vi "HapticSTM-Height.vi"() -> ()   [LabVIEW 2019]
uses:
  <userlib>/HapticSTM/HapticSTM.lvlib
panel:
  out "ZVAL":dbl
  out "Target Z":dbl
  out "Target X":dbl
  out "Z Out":dbl
  out "X Out":dbl
  out "Max speed":dbl
  out "FW":dbl
  out "VY":dbl
  out "VZ":dbl
  out "VX":dbl
  in  "Drag":dbl=1.0
  in  "STOP":bool
  in  "START":bool
  out "Fy":dbl
  out "Fz":dbl
  out "phi":dbl
  out "psi":dbl
  out "Fx":dbl
  out "theta":dbl
  out "x":dbl
  out "y":dbl
  out "z":dbl
  in  "Sensitivity":dbl=3.5
  out "Clicks":dbl
  out "Scope":dbl
  out "FH":dbl
  # "Sample Window"
  # "Position"
  # "Force"
  # "Angles"
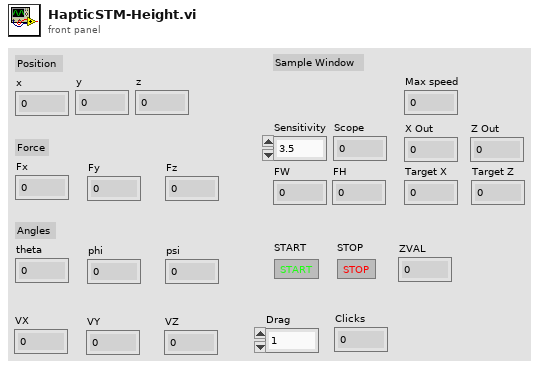
[diagram p1: front panel]
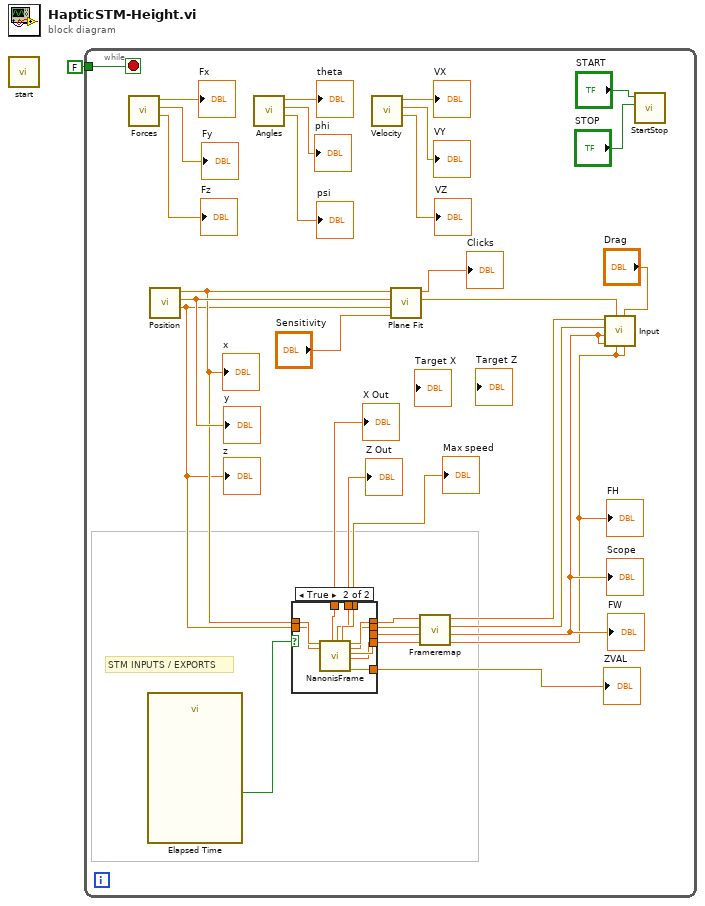
[diagram p0: block diagram]
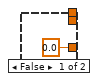
[diagram p2: hidden frame]
diagram:
  n1 = call <userlib>:"start.vi"() -> ()  [unwired: 11 in, 1 out]
  n2 = while {
    tunnel: FALSE -> [w21]
    stop <- w21 stop-if-true
    # "STM INPUTS / EXPORTS"
    n3 = call <userlib>:"Forces.vi"() -> ("Fz"=→"Fz":dbl, "Fy"=→"Fy":dbl, "Fx"=→"Fx":dbl)  [unwired: 9 in]
    n4 = call "Elapsed Time"() -> ("Time has Elapsed"=w3:bool)  [unwired: 12 in, 7 out]
    n5 = call <userlib>:"Position.vi"() -> ("Z"=w10:dbl, "Y"=w28:dbl, "X"=w11:dbl)  [unwired: 9 in]
    "x" <- w11
    "y" <- w28
    "z" <- w10
    n6 = call <userlib>:"Angles.vi"() -> ("psi"=→"psi":dbl, "phi"=→"phi":dbl, "theta"=→"theta":dbl)  [unwired: 9 in]
    n7 = case shown="True" w3 {
      tunnel: [_ w44] -> w12
      tunnel: w11 -> [_ w43]
      tunnel: w10 -> [_ w42]
      tunnel: [_ w41] -> w9
      tunnel: [_ w40] -> w8
      tunnel: [_ w39] -> w7
      tunnel: [_ w38] -> w6
      tunnel: [_ w37] -> w5
      tunnel: [_ w36] -> w4
      tunnel: [0.0 ("ZVAL") w35] -> w2
      frame False {
      }
      frame True {
        n8 = call <userlib>:"NanonisFrame.vi"("x"=w43, "z"=w42) -> ("X Out"=w37:dbl, "Z Out"=w36:dbl, "Speed"=w44:dbl, "FO X"=w41:dbl, "FO Z"=w40:dbl, "FW"=w39:dbl, "FH"=w38:dbl, "CVAL (nA)"=w35:dbl)  [unwired: 10 in]
      }
    }
    "Max speed" <- w12
    "Z Out" <- w4
    "X Out" <- w5
    "ZVAL" <- w2
    n9 = call <userlib>:"Velocity.vi"() -> ("VZ"=→"VZ":dbl, "VY"=→"VY":dbl, "VX"=→"VX":dbl)  [unwired: 9 in]
    n10 = call <userlib>:"Plane Fit.vi"("Sensitivity"="Sensitivity", "Z"=w10, "Nano Z"=w28, "X"=w11) -> ("Output"=w25:dbl, "Clicks"=→"Clicks":dbl)  [unwired: 6 in]
    n11 = call <userlib>:"Frameremap.vi"("FH"=w6, "FW"=w7, "FO Z"=w8, "FO X"=w9) -> ("FH"=w13:dbl, "FW"=w14:dbl, "Z Origin"=w23:dbl, "X Origin"=w24:dbl)  [unwired: 4 in]
    "Scope" <- w14
    "FH" <- w13
    "FW" <- w14
    n12 = call <userlib>:"Input.vi"("Scopez"=w13, "Drag"="Drag", "FH"=w13, "Signal in"=w25, "FW"=w14, "Scopex"=w14, "Z origin"=w23, "X origin"=w24) -> ()  [unwired: 3 in, 1 out]
    n13 = call <userlib>:"StartStop.vi"("STOP"="STOP", "START"="START") -> ()  [unwired: 10 in]
  }
